vi "Produce Display.vi"(0 "Channel Setting 2":T3(array[cluster])=[{"Channel"=1, "Gain"=1, "Shunt Resistor"=5, "Measure"=1}, {"Channel"=2, "Gain"=1, "Shunt Resistor"=5, "Measure"=1}, {"Channel"=3, "Gain"=1, "Shunt Resistor"=1, "Measure"=2}, {"Channel"=4, "Gain"=1, "Shunt Resistor"=1, "Measure"=2}] {"Measure" items=["Float", "Current(Diff)", "Voltage(SE+)"]; "Shunt Resistor" items=["Open"=1, "50 Ohms"=2, "500 Ohms"=3, "5k Ohms"=4, "50k Ohms"=5]; "Gain" items=["1x"=1, "10x"=2, "100x"=3, "1000x"=4]; "Channel" items=["Channel 1"=1, "Channel 2"=2, "Channel 3"=3, "Channel 4"=4, "Channel 5"=5, "Channel 6"=6, "Channel 7"=7, "Channel 8"=8]}, 1 "Demodulation In":dbl[][](array[numeric])=[[1.4839408729757508e-11, -1.900879392885926e-12, 1.4960661546706472e-11, -7.299647829275913], [1.7200124080450918e-16, -5.0346392409039706e-17, 1.7921826376487348e-16, -16.315253344298398], [1.1117395670783847e-11, -2.59351111233741e-11, 2.8217485279211652e-11, -66.79702725745167], [-3.930657765785384e-11, 1.8195590831737717e-12, 3.934867014817724e-11, 177.3495865094821]], 2 "Display":u16(ring) items=["X and Y", "R and Theta"], 3 "Input Signals In":i16(slide)=1 scale=1.0..20.0, 4 "Lockin Display A In":i16(slide)=1 scale=1.0..18.0, 5 "Lockin Display D In":i16(slide)=4 scale=1.0..18.0, 6 "Lockin Display C In":i16(slide)=3 scale=1.0..18.0, 7 "Lockin Display B In":i16(slide)=2 scale=1.0..18.0) -> (15 "Results":dbl[][](array[numeric])=[[1.1085752698169061e-06, 8.970523484593692e-07, 1.426058219262487e-06, 38.9795731407906], [0.009851325382064164, -0.0009794262328395094, 0.009899893308964286, -5.677731707079707], [1.3085970697368273e-06, 7.35860824175527e-07, 1.5013052466038e-06, 29.35026849878307], [2.653910755996262e-06, 1.0145343098285082e-06, 2.8412184299366806e-06, 20.9208047375633], [-6.086289413703597e-07, 1.180787094252328e-06, 1.3284153530528245e-06, 117.2685442231227], [2.777937660299593e-06, 8.877049230863689e-07, 2.9163260577278655e-06, 17.721560078700946]], 17 "Display Cluster (Not Into Cases) Out":T1, 18 "Display Cluster (Into Cases) Out cluster":T2)   [LabVIEW 2013, in "Lock-In Variable Channels_2.lvclass"]
uses:
  Lock-In Variable Channels_2.lvclass
panel:
  out "Gain":u16[](array[numeric])
  out "Measure?":u16[](array[numeric])
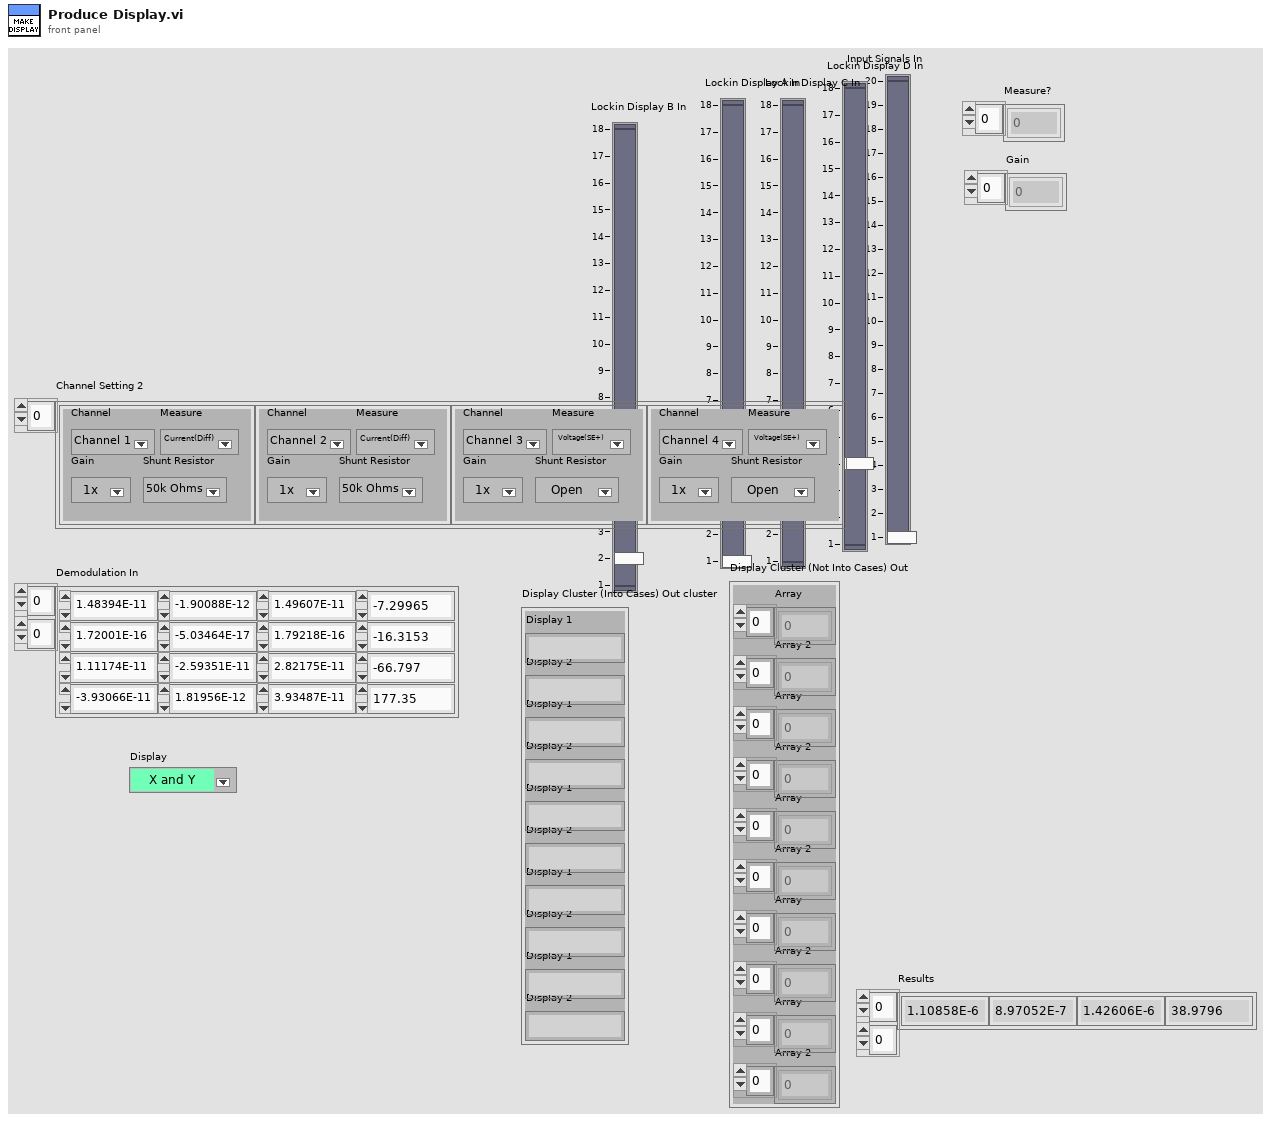
[diagram p1: front panel]
types:
  T1 = cluster{"Array":dbl[], "Array 2":dbl[], "Array":dbl[], "Array 2":dbl[], "Array":dbl[], "Array 2":dbl[], "Array":dbl[], "Array 2":dbl[], "Array":dbl[], "Array 2":dbl[]}
  T2 = cluster{"Display 1":string, "Display 2":string, "Display 1":string, "Display 2":string, "Display 1":string, "Display 2":string, "Display 1":string, "Display 2":string, "Display 1":string, "Display 2":string}
  T3 = cluster{"Channel":u16, "Gain":u16, "Shunt Resistor":u16, "Measure":u16}[]
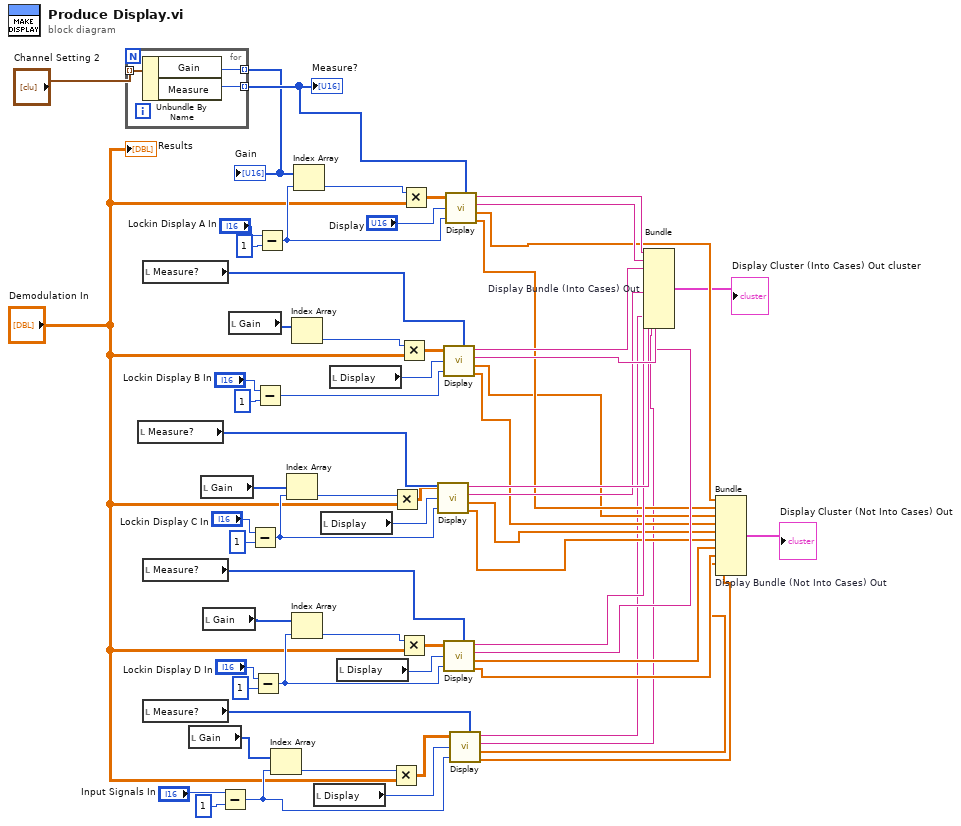
[diagram p0: block diagram]
diagram:
  n1 = for {
    tunnel: "Channel Setting 2" -> [w67] mode=indexing
    tunnel: [w66] -> w63 mode=indexing
    tunnel: [w65] -> w64 mode=indexing
    n2 = Unbundle By Name(w67) -> ("Gain"=w66:u16, "Measure"=w65:u16)
  }
  "Gain" <- w63
  "Measure?" <- w64
  n3 = local read "Measure?"() -> (w44:u16[])
  n4 = local read "Measure?"() -> (w45:u16[])
  n5 = local read "Measure?"() -> (w43:u16[])
  n6 = local read "Measure?"() -> (w56:u16[])
  n7 = local read "Gain"() -> (w55:u16[])
  n8 = local read "Gain"() -> (w47:u16[])
  n9 = local read "Gain"() -> (w48:u16[])
  n10 = Subtract(x="Input Signals In", y=i16 1) -> (x-y=w61:i16)
  n11 = local read "Gain"() -> (w46:u16[])
  n12 = Subtract(x="Lockin Display C In", y=i16 1) -> (x-y=w38:i16)
  n13 = Subtract(x="Lockin Display D In", y=i16 1) -> (x-y=w39:i16)
  n14 = Subtract(x="Lockin Display B In", y=i16 1) -> (x-y=w31:i16)
  n15 = Subtract(x="Lockin Display A In", y=i16 1) -> (x-y=w30:i16)
  n16 = Index Array(array=w55, index=w61) -> (element=w57:u16)
  n17 = Index Array(array=w47, index=w38) -> (element=w37:u16)
  n18 = Index Array(array=w46) -> (element=w32:u16)  [unwired: 1 in]
  n19 = Index Array(array=w48, index=w39) -> (element=w40:u16)
  n20 = Index Array(array=w63, index=w30) -> (element=w29:u16)
  n21 = local read "Display"() -> (w59:u16)
  n22 = local read "Display"() -> (w50:u16)
  n23 = local read "Display"() -> (w49:u16)
  n24 = local read "Display"() -> (w51:u16)
  n25 = Multiply(x=w57, y="Demodulation In") -> (x*y=w58:dbl[][])
  n26 = Multiply(x=w37, y="Demodulation In") -> (x*y=w36:dbl[][])
  n27 = Multiply(x=w32, y="Demodulation In") -> (x*y=w33:dbl[][])
  n28 = Multiply(x=w40, y="Demodulation In") -> (x*y=w41:dbl[][])
  n29 = Multiply(x=w29, y="Demodulation In") -> (x*y=w28:dbl[][])
  n30 = call "Display.vi"("Results"=w36, "Display"=w50, "Lock-in #"=w38, "Amplifier Settings"=w44) -> ("Display 1"=w18:string, "Display 2"=w17:string, "Array"=w10:dbl[], "Array 2"=w9:dbl[])  [unwired: 3 in]
  n31 = call "Display.vi"("Results"=w33, "Display"=w49, "Lock-in #"=w31, "Amplifier Settings"=w45) -> ("Display 1"=w20:string, "Display 2"=w19:string, "Array"=w12:dbl[], "Array 2"=w11:dbl[])  [unwired: 3 in]
  n32 = call "Display.vi"("Results"=w41, "Display"=w51, "Lock-in #"=w39, "Amplifier Settings"=w43) -> ("Display 1"=w16:string, "Display 2"=w15:string, "Array"=w8:dbl[], "Array 2"=w7:dbl[])  [unwired: 3 in]
  n33 = call "Display.vi"("Results"=w28, "Display"="Display", "Lock-in #"=w30, "Amplifier Settings"=w64) -> ("Display 1"=w22:string, "Display 2"=w21:string, "Array"=w14:dbl[], "Array 2"=w13:dbl[])  [unwired: 3 in]
  n34 = call "Display.vi"("Results"=w58, "Display"=w59, "Lock-in #"=w61, "Amplifier Settings"=w56) -> ("Display 1"=w3:string, "Display 2"=w2:string, "Array"=w5:dbl[], "Array 2"=w4:dbl[])  [unwired: 3 in]
  n35 = Bundle "Display Bundle (Into Cases) Out"("Display 1"=w22, "Display 2"=w21, "Display 1"=w20, "Display 2"=w19, "Display 1"=w18, "Display 2"=w17, "Display 1"=w16, "Display 2"=w15, "Display 1"=w3, "Display 2"=w2) -> (→"Display Cluster (Into Cases) Out cluster":T2)  [unwired: 1 in]
  n36 = Bundle "Display Bundle (Not Into Cases) Out"("Array"=w14, "Array 2"=w13, "Array"=w12, "Array 2"=w11, "Array"=w10, "Array 2"=w9, "Array"=w8, "Array 2"=w7, "Array"=w5, "Array 2"=w4) -> (→"Display Cluster (Not Into Cases) Out":T1)  [unwired: 1 in]
  "Results" <- "Demodulation In"
